vi "MemoryToLvData_PTR.vi"(7 "Type":variant, 8 "error in (no error)":errorcluster, 10 "ByteArray":u8[](array[numeric])) -> (0 "error out":errorcluster, 1 "Supported Type?":bool, 2 "data":variant, 4 "ByteArray Left":u8[](array[numeric]))   [LabVIEW 2019, in "Memory Data Access.lvlib"]
uses:
  Memory Data Access.lvlib
  <vilib>/Utility/Data Type/Type Definitions/Data Type.ctl
  Typedef/memoryDataBlock.ctl
  Global/Global.vi
  <vilib>/Utility/Data Type/NI_Data Type.lvlib
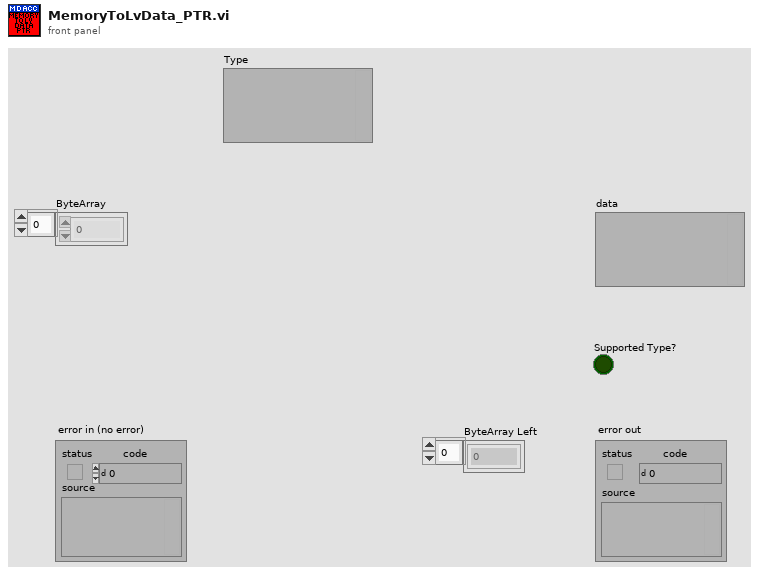
[diagram p1: front panel]
types:
  T1 = typedef "NI_Data Type.lvlib/Data Type.ctl" = enum8{"Invalid Type", "Void", "I8", "I16", "I32", "I64", "U8", "U16", "U32", "U64", "Single Float", "Double Float", "Extended Float", "Single Complex", "Double Complex", "Extended Complex", "Enum U8", "Enum U16", "Enum U32", "Enum U64", "Single Float With Unit", "Double Float With Unit", "Extended Float With Unit", "Single Complex with Unit", "Double Complex with Unit", "Extended Complex with Unit", "Boolean", "String", "Path", "Picture", "Tag", "Array", "Cluster", "Variant", "LV Variant", "Waveform", "Timestamp", "Digital Waveform", "Digital Data", "ExpressData", "Refnum", "External Data", "VI", "Poly VI", "LabVIEW Class Instance", "Fixed Point", "Set Collection", "Map Collection"}
  T2 = typedef "Memory Data Access.lvlib/memoryDataBlock.ctl" = cluster{"Length":u32, "Addr":u64}
  T3 = typedef "Type Descriptor Enumeration__ogtk.ctl" = enum8{"<Null>", "I8", "I16", "I32", "I64", "U8", "U16", "U32", "U64", "SGL", "DBL", "EXT", "CSG", "CDB", "CXT", "0x0F", "0x10", "0x11", "0x12", "0x13", "0x14", "Enum U8", "Enum U16", "Enum U32", "Enum U64", "SGL PQ", "DBL PQ", "EXT PQ", "CSG PQ", "CDB PQ", "CXT PQ", "0x1F", "0x20", "Boolean", "0x22", "0x23", "0x24", "0x25", "0x26", "0x27", "0x28", "0x29", "0x2A", "0x2B", "0x2C", "0x2D", "0x2E", "0x2F", "String", "0x31", "Path", "Pict", "0x34", "0x35", "0x36", "DAQ", "0x38", "0x39", "0x3A", "0x3B", "0x3C", "0x3D", "0x3E", "0x3F", "Array", "0x41", "0x42", "0x43", "0x44", "0x45", "0x46", "0x47", "0x48", "0x49", "0x4A", "0x4B", "0x4C", "0x4D", "0x4E", "0x4F", "Cluster", "0x51", "0x52", "Variant", "Waveform", "0x55", "0x56", "0x57", "0x58", "0x59", "0x5A", "0x5B", "0x5C", "0x5D", "0x5E", "0x5F", "0x60", "0x61", "0x62", "0x63", "0x64", "0x65", "0x66", "0x67", "0x68", "0x69", "0x6A", "0x6B", "0x6C", "0x6D", "0x6E", "0x6F", "Refnum"}
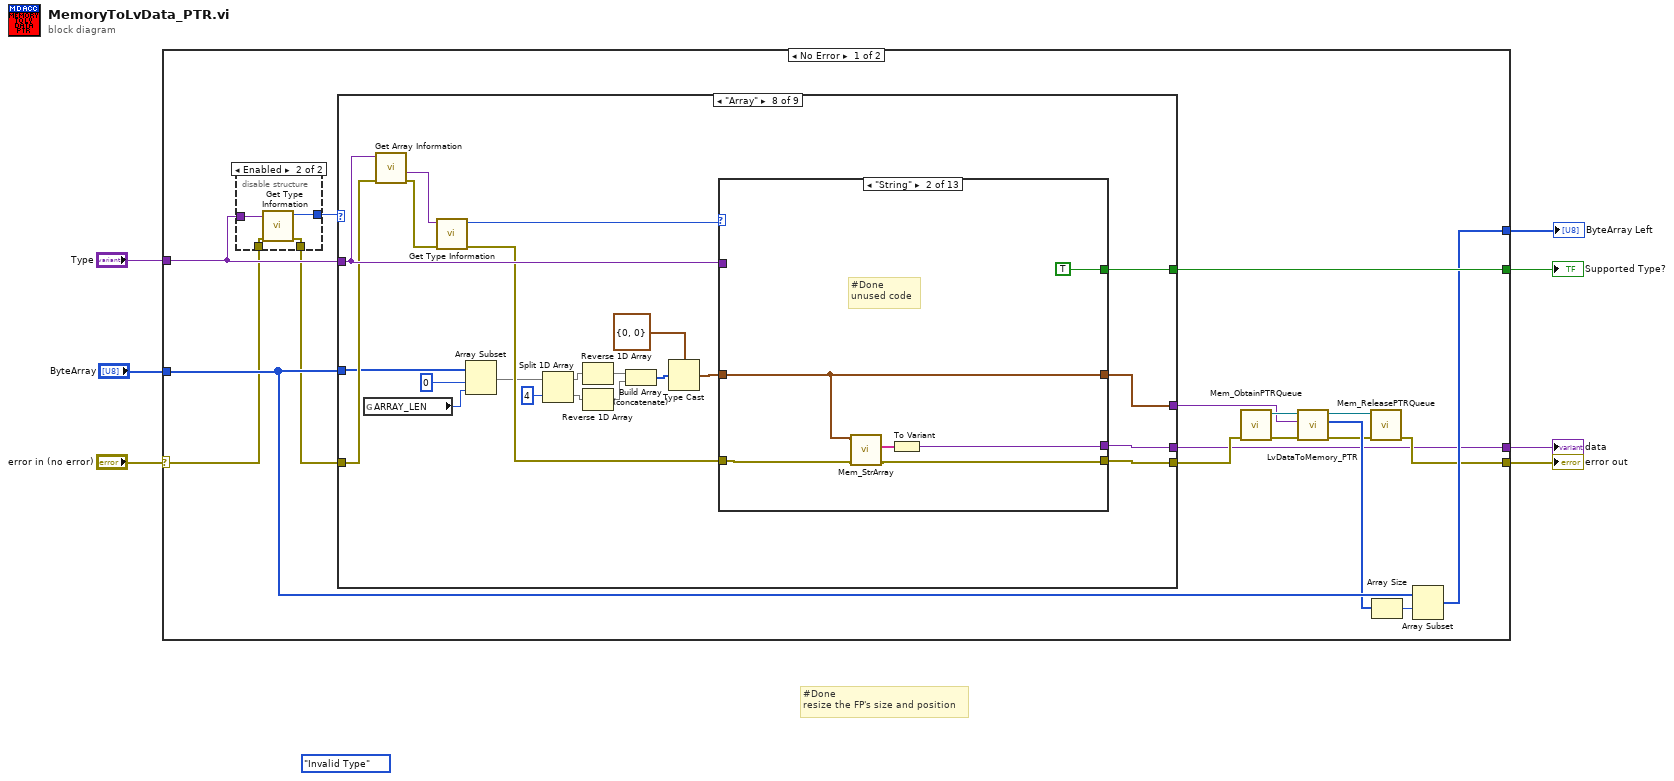
[diagram p0: block diagram]
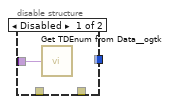
[diagram p2: hidden frame]
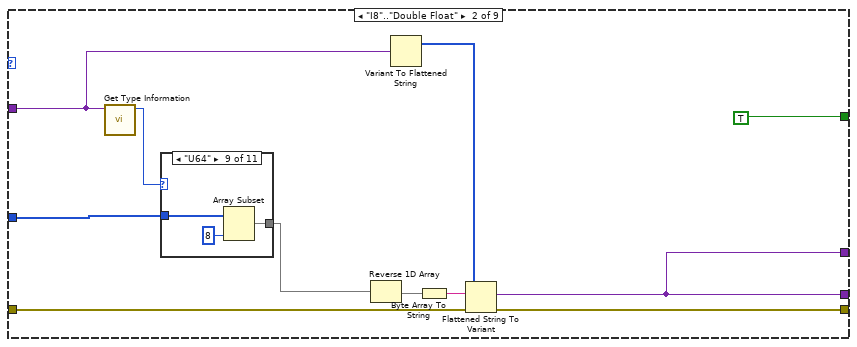
[diagram p4: hidden frame]
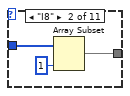
[diagram p6: hidden frame]
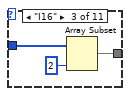
[diagram p7: hidden frame]
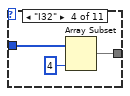
[diagram p8: hidden frame]
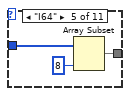
[diagram p9: hidden frame]
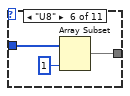
[diagram p10: hidden frame]
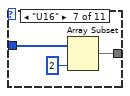
[diagram p11: hidden frame]
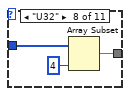
[diagram p12: hidden frame]
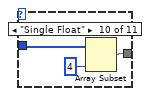
[diagram p13: hidden frame]
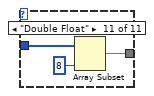
[diagram p14: hidden frame]
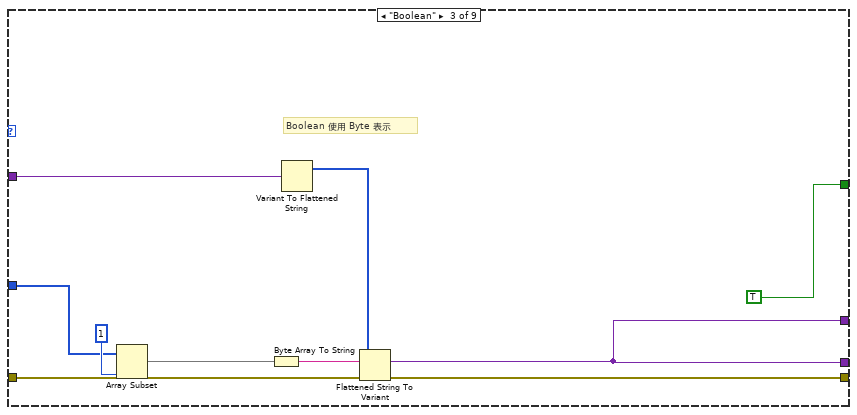
[diagram p15: hidden frame]
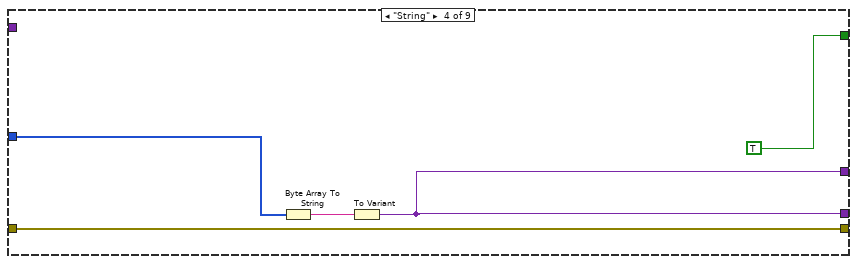
[diagram p16: hidden frame]
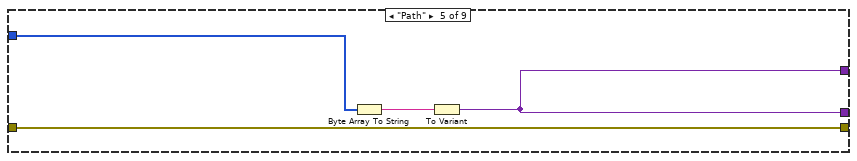
[diagram p17: hidden frame]
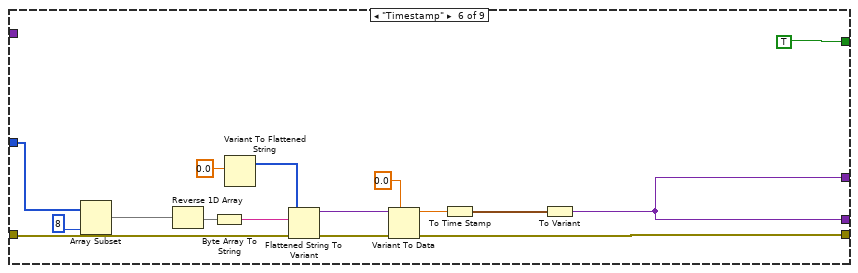
[diagram p18: hidden frame]
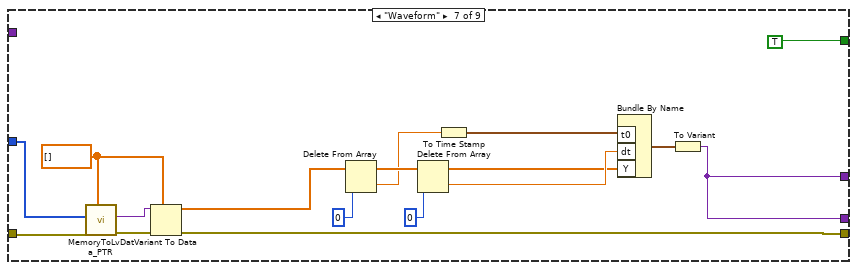
[diagram p19: hidden frame]
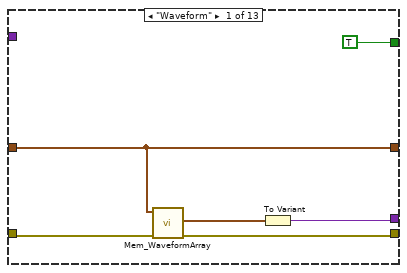
[diagram p20: hidden frame]
diagram:
  (unwired) Data_Type."Invalid Type" ("type")
  # "#Done\nresize the FP's size and position"
  n1 = case shown="No Error" "error in (no error)" {
    selector: "error in (no error)" -> [w17 w243]
    tunnel: "ByteArray" -> [w22 _]
    tunnel: [w10 w243] -> w5
    tunnel: "Type" -> [w24 _]
    tunnel: [w9 _] -> w3
    tunnel: [w23 _] -> w2
    tunnel: [w21 _] -> w1
    frame No Error {
      n2 = disable-structure shown="Enabled" {
        disable-tunnel: w24 -> [w25 w30]
        disable-tunnel: [_ w29] -> w18
        disable-tunnel: w17 -> [_ w28]
        disable-tunnel: [_ w27] -> w16
        frame Disabled {
          n3 = call <userlib>:"Get TDEnum from Data__ogtk.vi"("Data"=w25) -> ("Type Descriptor Enumeration"=w26:T3)  [unwired: 4 in]
        }
        frame Enabled {
          n4 = call <vilib>:"Get Type Information.vi"("error in (no error)"=w28, "variant"=w30) -> ("error out"=w27:errorcluster, "type"=w29:T1)  [unwired: 5 in, 3 out]
        }
      }
      n5 = case shown="\"Array\"" w18 {
        tunnel: w16 -> [w32 w37 w81 w87 w92 w106 w125 w147 w225]
        tunnel: [w32 w41 w80 w87 w92 w99 w124 w146 w227] -> w14
        tunnel: w24 -> [w31 w34 w83 _ _ _ _ w148 w230]
        tunnel: [_ TRUE TRUE TRUE _ TRUE TRUE w142 w233] -> w23
        tunnel: w22 -> [_ w36 w77 w88 w93 w96 w122 w141 w231]
        tunnel: [w31 w33 w75 w85 w90 w94 w110 w135 w222] -> w8
        tunnel: [_ w33 w75 w85 w90 w94 w110 w134 w222] -> w9
        frame "Invalid Type", Default {
        }
        frame "I8".."Double Float" {
          n6 = call <vilib>:"Get Type Information.vi"("variant"=w34) -> ("type"=w38:T1)  [unwired: 6 in, 4 out]
          n7 = case shown="\"U64\"" w38 {
            tunnel: w36 -> [w44 w47 w49 w52 w55 w58 w61 w64 w67 w70 w73]
            tunnel: [w44 w45 w48 w51 w54 w57 w60 w63 w66 w69 w72] -> w35
            frame "Invalid Type", Default {
            }
            frame "I8" {
              n8 = Array Subset(array=w47, length=1) -> (w45:u8[])  [unwired: 1 in]
            }
            frame "I16" {
              n9 = Array Subset(array=w49, length=2) -> (w48:u8[])  [unwired: 1 in]
            }
            frame "I32" {
              n10 = Array Subset(array=w52, length=4) -> (w51:u8[])  [unwired: 1 in]
            }
            frame "I64" {
              n11 = Array Subset(array=w55, length=8) -> (w54:u8[])  [unwired: 1 in]
            }
            frame "U8" {
              n12 = Array Subset(array=w58, length=1) -> (w57:u8[])  [unwired: 1 in]
            }
            frame "U16" {
              n13 = Array Subset(array=w61, length=2) -> (w60:u8[])  [unwired: 1 in]
            }
            frame "U32" {
              n14 = Array Subset(array=w64, length=4) -> (w63:u8[])  [unwired: 1 in]
            }
            frame "U64" {
              n15 = Array Subset(array=w67, length=8) -> (w66:u8[])  [unwired: 1 in]
            }
            frame "Single Float" {
              n16 = Array Subset(array=w70, length=4) -> (w69:u8[])  [unwired: 1 in]
            }
            frame "Double Float" {
              n17 = Array Subset(array=w73, length=8) -> (w72:u8[])  [unwired: 1 in]
            }
          }
          n18 = Reverse 1D Array(array=w35) -> (reversed array=w39:u8[])
          n19 = Variant To Flattened String(Variant=w34) -> (1:w42:i16[])  [unwired: 1 out]
          n20 = Byte Array To String(unsigned byte array=w39) -> (string=w40:string)
          n21 = Flattened String To Variant(4:w37, 6:w40, 7:w42) -> (0:w41:errorcluster, 3:w33:variant)
        }
        frame "Boolean" {
          # "Boolean 使用 Byte 表示"
          n22 = Array Subset(array=w77, length=1) -> (w76:u8[])  [unwired: 1 in]
          n23 = Byte Array To String(unsigned byte array=w76) -> (string=w79:string)
          n24 = Variant To Flattened String(Variant=w83) -> (1:w82:i16[])  [unwired: 1 out]
          n25 = Flattened String To Variant(4:w81, 6:w79, 7:w82) -> (0:w80:errorcluster, 3:w75:variant)
        }
        frame "String" {
          n26 = Byte Array To String(unsigned byte array=w88) -> (string=w86:string)
          n27 = To Variant(anything=w86) -> (Variant=w85:variant)
        }
        frame "Path" {
          n28 = Byte Array To String(unsigned byte array=w93) -> (string=w91:string)
          n29 = To Variant(anything=w91) -> (Variant=w90:variant)
        }
        frame "Timestamp" {
          n30 = Array Subset(array=w96, length=8) -> (w95:u8[])  [unwired: 1 in]
          n31 = Reverse 1D Array(array=w95) -> (reversed array=w107:u8[])
          n32 = Byte Array To String(unsigned byte array=w107) -> (string=w108:string)
          n33 = Variant To Flattened String(Variant=0.0) -> (1:w109:i16[])  [unwired: 1 out]
          n34 = Flattened String To Variant(4:w106, 6:w108, 7:w109) -> (0:w103:errorcluster, 3:w104:variant)
          n35 = Variant To Data(error in=w103, type=0.0, Variant=w104) -> (data=w101:dbl, error out=w99:errorcluster)
          n36 = To Time Stamp(1:w101) -> (0:w100:timestamp)
          n37 = To Variant(anything=w100) -> (Variant=w94:variant)
        }
        frame "Waveform" {
          w111 = dbl[] [] ("array")
          n38 = call "MemoryToLvData_PTR.vi"("Type"=w111, "error in (no error)"=w125, "ByteArray"=w122) -> ("error out"=w113:errorcluster, "data"=w114:variant)  [unwired: 5 in, 2 out]
          n39 = Variant To Data(error in=w113, type=w111, Variant=w114) -> (data=w112:dbl[], error out=w124:errorcluster)
          n40 = Delete From Array(array=w112, index=0) -> (deleted portion=w118:dbl, array with subset deleted=w121:dbl[])  [unwired: 1 in]
          n41 = Delete From Array(array=w121, index=0) -> (deleted portion=w116:dbl, array with subset deleted=w115:dbl[])  [unwired: 1 in]
          n42 = To Time Stamp(1:w118) -> (0:w117:timestamp)
          n43 = Bundle By Name("t0"=w117, "dt"=w116, "Y"=w115) -> (w123:waveform(dbl))  [unwired: 1 in]
          n44 = To Variant(anything=w123) -> (Variant=w110:variant)
        }
        frame "Array" {
          n45 = global read "Global.vi" "ARRAY_LEN"() -> (w139:u32)
          n46 = call <vilib>:"Get Array Information.vi"("error in (no error)"=w147, "variant"=w148) -> ("error out"=w143:errorcluster, "array element data type"=w145:variant)  [unwired: 6 in, 2 out]
          n47 = call <vilib>:"Get Type Information.vi"("error in (no error)"=w143, "variant"=w145) -> ("error out"=w136:errorcluster, "type"=w144:T1)  [unwired: 5 in, 3 out]
          n48 = Array Subset(array=w141, index=0, length=w139) -> (w133:u8[])
          n49 = Split 1D Array(array=w133, index=4) -> (first subarray=w131:u8[], second subarray=w130:u8[])
          n50 = Reverse 1D Array(array=w131) -> (reversed array=w129:u8[])
          n51 = Reverse 1D Array(array=w130) -> (reversed array=w128:u8[])
          n52 = Build Array (concatenate)(w129, w128) -> (w127:u8[])
          n53 = Type Cast(type=T2 {"Length"=0, "Addr"=0} ("dataInfo"), x=w127) -> (*(type *) &x=w137:T2)
          n54 = case shown="\"String\"" w144 {
            tunnel: w148 -> [_ _ _ _ _ _ _ _ _ _ _ _ _]
            tunnel: w136 -> [w153 w159 w165 w171 w177 w179 w184 w190 w196 w202 w208 w214 w219]
            tunnel: [w152 w158 w164 w170 w176 w179 w183 w189 w195 w201 w207 w213 w218] -> w146
            tunnel: [TRUE TRUE TRUE TRUE TRUE _ TRUE TRUE TRUE TRUE TRUE TRUE TRUE] -> w142
            tunnel: w137 -> [w151 w157 w163 w169 w175 _ w182 w188 w194 w200 w206 w212 w220]
            tunnel: [w151 w157 w163 w169 w175 _ w182 w188 w194 w200 w206 w212 w220] -> w135
            tunnel: [w149 w155 w161 w167 w173 _ w180 w187 w193 w199 w204 w211 w216] -> w134
            frame "Waveform" {
              n55 = call "Mem_WaveformArray.vi"("error in (no error)"=w153, "dataInfo"=w151) -> ("error out"=w152:errorcluster, "Array"=w150:waveform(dbl)[])  [unwired: 8 in]
              n56 = To Variant(anything=w150) -> (Variant=w149:variant)
            }
            frame "String" {
              # "#Done\nunused code"
              n57 = call "Mem_StrArray.vi"("error in (no error)"=w159, "dataInfo"=w157) -> ("error out"=w158:errorcluster, "SreArray"=w156:string[])  [unwired: 8 in]
              n58 = To Variant(anything=w156) -> (Variant=w155:variant)
            }
            frame "I8" {
              n59 = call "Mem_I8Array.vi"("error in (no error)"=w165, "dataInfo"=w163) -> ("error out"=w164:errorcluster, "DataPoints"=w162:i8[])  [unwired: 8 in]
              n60 = To Variant(anything=w162) -> (Variant=w161:variant)
            }
            frame "I16" {
              n61 = call "Mem_I16Array.vi"("error in (no error)"=w171, "dataInfo"=w169) -> ("error out"=w170:errorcluster, "DataPoints"=w168:i16[])  [unwired: 8 in]
              n62 = To Variant(anything=w168) -> (Variant=w167:variant)
            }
            frame "I32" {
              n63 = call "Mem_I32Array.vi"("error in (no error)"=w177, "dataInfo"=w175) -> ("error out"=w176:errorcluster, "DataPoints"=w174:i32[])  [unwired: 8 in]
              n64 = To Variant(anything=w174) -> (Variant=w173:variant)
            }
            frame "Invalid Type", Default {
            }
            frame "I64" {
              n65 = call "Mem_I64Array.vi"("error in (no error)"=w184, "dataInfo"=w182) -> ("error out"=w183:errorcluster, "DataPoints"=w181:i64[])  [unwired: 8 in]
              n66 = To Variant(anything=w181) -> (Variant=w180:variant)
            }
            frame "U8" {
              n67 = call "Mem_U8Array.vi"("error in (no error)"=w190, "dataInfo"=w188) -> ("error out"=w189:errorcluster, "DataPoints"=w186:u8[])  [unwired: 8 in]
              n68 = To Variant(anything=w186) -> (Variant=w187:variant)
            }
            frame "U16" {
              n69 = call "Mem_U16Array.vi"("error in (no error)"=w196, "dataInfo"=w194) -> ("error out"=w195:errorcluster, "DataPoints"=w192:u16[])  [unwired: 8 in]
              n70 = To Variant(anything=w192) -> (Variant=w193:variant)
            }
            frame "U32" {
              n71 = call "Mem_U32Array.vi"("error in (no error)"=w202, "dataInfo"=w200) -> ("error out"=w201:errorcluster, "DataPoints"=w198:u32[])  [unwired: 8 in]
              n72 = To Variant(anything=w198) -> (Variant=w199:variant)
            }
            frame "U64" {
              n73 = call "Mem_U64Array.vi"("error in (no error)"=w208, "dataInfo"=w206) -> ("error out"=w207:errorcluster, "DataPoints"=w205:u64[])  [unwired: 8 in]
              n74 = To Variant(anything=w205) -> (Variant=w204:variant)
            }
            frame "Single Float" {
              n75 = call "Mem_SGLArray.vi"("error in (no error)"=w214, "dataInfo"=w212) -> ("error out"=w213:errorcluster, "DataPoints"=w210:sgl[])  [unwired: 8 in]
              n76 = To Variant(anything=w210) -> (Variant=w211:variant)
            }
            frame "Double Float" {
              n77 = call "Mem_DBLArray.vi"("error in (no error)"=w219, "dataInfo"=w220) -> ("error out"=w218:errorcluster, "DataPoints"=w217:dbl[])  [unwired: 8 in]
              n78 = To Variant(anything=w217) -> (Variant=w216:variant)
            }
          }
        }
        frame "Cluster" {
          n79 = call <userlib>:"Get Data Name__ogtk.vi"("error in (no error)"=w225, "Data"=w230) -> ("error out"=w226:errorcluster, "Data Name"=w224:string, "Data dup"=w223:variant)  [unwired: 7 in]
          n80 = call <userlib>:"Cluster to Array of VData__ogtk.vi"("error in (no error)"=w226, "Cluster"=w223) -> ("error out"=w232:errorcluster, "Array of VData"=w235:variant[])  [unwired: 8 in]
          n81 = for {
            tunnel: w235 -> [w238] mode=indexing
            tunnel: [w241] -> w234 mode=indexing
            shift-right: [w242] -> w228
            shift-left: w232 -> [w236]
            shift-right: [w239] -> _
            shift-left: w231 -> [w237]
            tunnel: [w240] -> w229 mode=indexing
            n82 = call "MemoryToLvData_PTR.vi"("Type"=w238, "error in (no error)"=w236, "ByteArray"=w237) -> ("error out"=w242:errorcluster, "Supported Type?"=w241:bool, "data"=w240:variant, "ByteArray Left"=w239:u8[])  [unwired: 5 in]
          }
          n83 = call <userlib>:"Array of VData to VCluster__ogtk.vi"("error in (no error)"=w228, "Cluster Name"=w224, "Array"=w229) -> ("error out"=w227:errorcluster, "VCluster"=w222:variant)  [unwired: 7 in]
          n84 = And Array Elements(Boolean array=w234) -> (logical AND=w233:bool)
        }
      }
      n85 = call "Mem_ObtainPTRQueue.vi"("error in (no error)"=w14) -> ("error out"=w15:errorcluster, "queue out"=w13:refnum<queue>)  [unwired: 9 in]
      n86 = call "LvDataToMemory_PTR.vi"("error in (no error)"=w15, "Payload"=w8, "AddrQueueIn"=w13) -> ("error out"=w12:errorcluster, "ByteArray"=w20:u8[], "AddrQueueOut"=w11:refnum<queue>)  [unwired: 5 in, 1 out]
      n87 = call "Mem_ReleasePTRQueue.vi"("error in (no error)"=w12, "AddrQueueIn"=w11) -> ("error out"=w10:errorcluster)  [unwired: 9 in]
      n88 = Array Size(array=w20) -> (size(s)=w19:i32)
      n89 = Array Subset(array=w22, index=w19) -> (w21:u8[])  [unwired: 1 in]
    }
    frame Error {
    }
  }
  "error out" <- w5
  "data" <- w3
  "Supported Type?" <- w2
  "ByteArray Left" <- w1
